vi "Trav_cluster_Convert.vi"(4 "Traverse line in":T1 {"Carrier_2 Q (l/min)" format="%#.2f"; "Row Duration (mins)" format="%#.1f"; "Row No" min=0; "Trace Gas Concentration (%)" min=0.0 format="%#_4f"; "Carrier_1 Q (l/min)" format="%#.4f"; "Start X" format="%#.2f"; "Start Y" format="%#.2f"; "Start Z" format="%#.2f"; "End X" format="%#.2f"; "End Y" format="%#.2f"; "End Z" format="%#.2f"; "Tunnel Speed" format="%#.2f"; "Averaging time (mins)" min=0.0 format="%#.2f"}, 5 "Channel Values In":string[](array[string]), 6 "Row Number":i32, 7 "Channel names":string[](array[string])) -> (0 "Traverse line Out":T1 {"Carrier_2 Q (l/min)" format="%#.2f"; "Row Duration (mins)" format="%#.1f"; "Row No" min=0; "Trace Gas Concentration (%)" min=0.0 format="%#_4f"; "Carrier_1 Q (l/min)" format="%#.4f"; "Start X" format="%#.2f"; "Start Y" format="%#.2f"; "Start Z" format="%#.2f"; "End X" format="%#.2f"; "End Y" format="%#.2f"; "End Z" format="%#.2f"; "Tunnel Speed" format="%#.2f"; "Averaging time (mins)" min=0.0 format="%#.2f"})   [LabVIEW 2020]
uses:
  Traverse_cluster.ctl
  Spacing.ctl
  Controls/Multi_run_mode.ctl
panel:
  # "X           Y          Z"
  # "Start"
  # "End"
  # "X           Y          Z"
  # "Start"
  # "End"
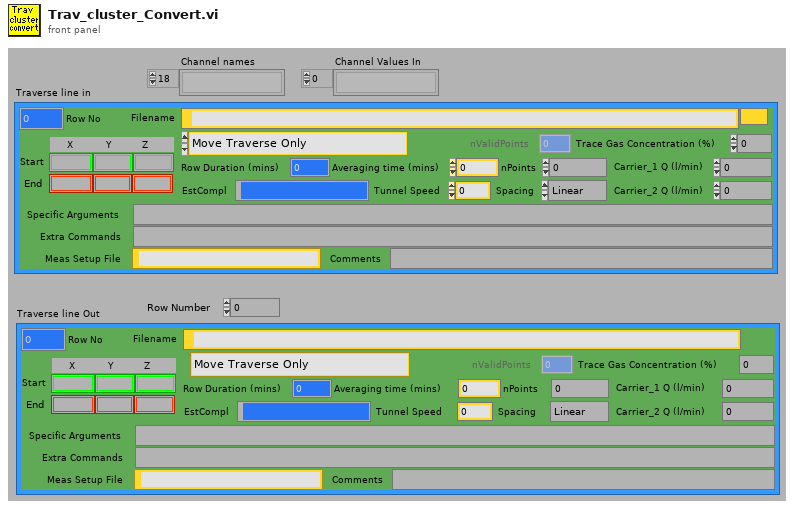
[diagram p1: front panel]
types:
  T1 = typedef "Traverse_cluster.ctl" = cluster{"Start X":sgl, "Start Y":sgl, "Start Z":sgl, "End X":sgl, "End Y":sgl, "End Z":sgl, "nPoints":i32, "Spacing":T2, "Filename":path, "Tunnel Speed":dbl, "Averaging time (mins)":dbl, "Extra Commands":string, "Carrier_1 Q (l/min)":dbl, "Carrier_2 Q (l/min)":dbl, "Trace Gas Concentration (%)":dbl, "Specific Arguments":string, "Comments":string, "Row No":i32, "Row Type Selector":T3, "EstCompl":string, "Row Duration (mins)":dbl, "nValidPoints":i32, "Meas Setup File":string}
  T2 = typedef "Spacing.ctl" = enum16{"Linear", "Log", "Gauss", "Specified", "N/A"}
  T3 = typedef "Multi_run_mode.ctl" = enum16{"Move Traverse Only", "Set Tunnel Speed Only", "Set Source Only", "Set Measurement Conditions", "Single Measurement", "Vertical Profile", "Lateral Profile", "Longitudinal Profile", "Multi-Axis Profile", "Explore Volume", "Auto Calibrate", "Meas Fast FID Bkgnd", "Check Beam Power", "Scanning Valve Measurement", "Run VI Named:", "Set ADAM Ch", "Wait (minutes)", "Send Message", "Synchronize With:", "Fall Back to this Row", "Turn Off Row Repeating", "Traverse 3D Volume", "Blank Row", "Jump to Fall Back Row"}
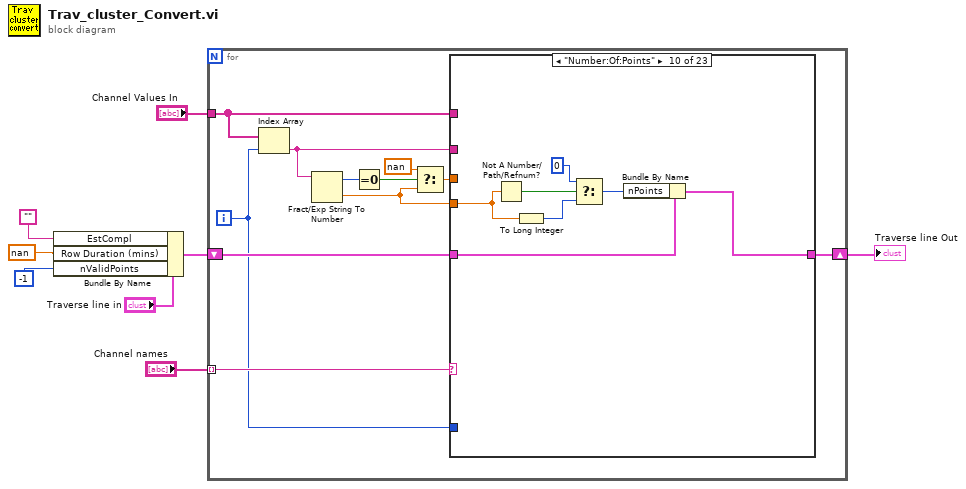
[diagram p0: block diagram]
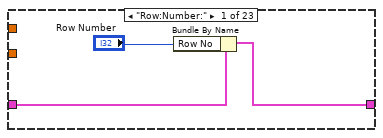
[diagram p2: hidden frame]
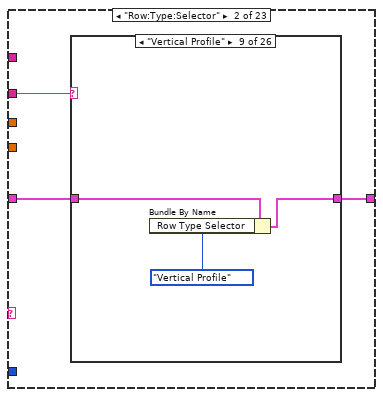
[diagram p3: hidden frame]
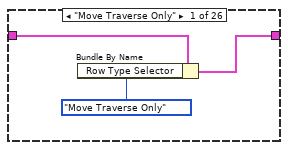
[diagram p4: hidden frame]
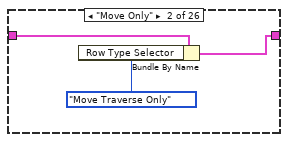
[diagram p5: hidden frame]
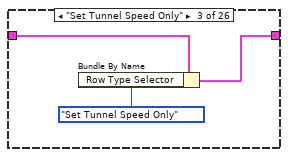
[diagram p6: hidden frame]
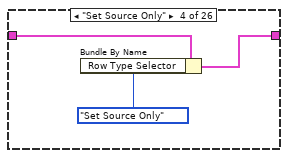
[diagram p7: hidden frame]
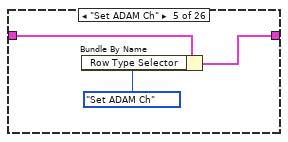
[diagram p8: hidden frame]
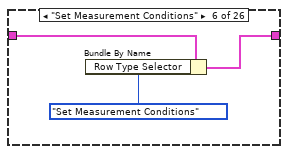
[diagram p9: hidden frame]
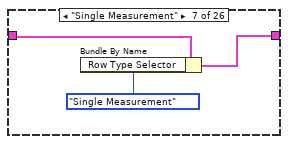
[diagram p10: hidden frame]
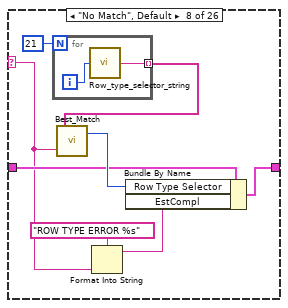
[diagram p11: hidden frame]
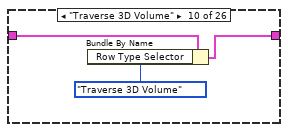
[diagram p12: hidden frame]
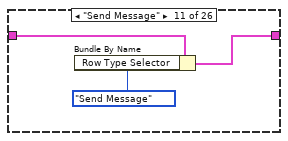
[diagram p13: hidden frame]
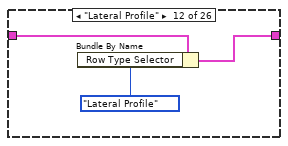
[diagram p14: hidden frame]
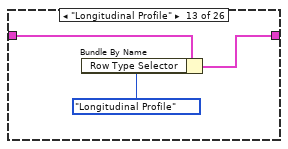
[diagram p15: hidden frame]
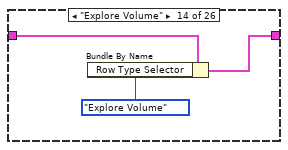
[diagram p16: hidden frame]
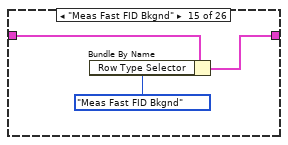
[diagram p17: hidden frame]
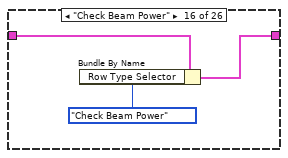
[diagram p18: hidden frame]
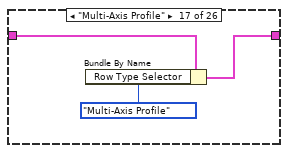
[diagram p19: hidden frame]
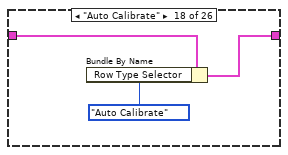
[diagram p20: hidden frame]
diagram:
  n1 = Bundle By Name(cluster="Traverse line in", "EstCompl"="", "Row Duration (mins)"=nan ("Bundle Element"), "nValidPoints"=-1 ("No. of Valid pts.")) -> (w4:T1)
  n2 = for {
    tunnel: "Channel names" -> [w13] mode=indexing
    shift-right: [w18] -> w3
    shift-left: w4 -> [w19]
    tunnel: "Channel Values In" -> [w10]
    i -> [w11]
    n3 = Index Array(array=w10, index=w11) -> (element=w12:string)
    n4 = Fract/Exp String To Number(string=w12) -> (offset past number=w17:i32, number=w9:dbl)  [unwired: 1 in, 2 out]
    n5 = Equal To 0?(x=w17) -> (x = 0?=w16:bool)
    n6 = Select(t=nan ("f"), s=w16, f=w9) -> (s? t:f=w15:dbl)
    n7 = case shown="\"Number:Of:Points\"" w13 {
      selector: w13 -> [_ _ _ _ _ _ _ _ _ _ _ _ _ _ _ _ _ _ _ _ _ _ w184]
      tunnel: w19 -> [w21 w24 w112 w115 w118 w122 w125 w127 w130 w132 w142 w148 w151 w156 w160 w163 w164 w167 w170 w176 w182 w183 w185]
      tunnel: w9 -> [_ _ _ _ _ _ _ _ _ w135 _ w147 _ _ _ _ w166 w169 w172 _ _ _ _]
      tunnel: [w22 w23 w113 w116 w119 w121 w124 w128 w131 w138 w141 w149 w154 w157 w159 w162 w165 w168 w171 w178 w182 w183 w185] -> w18
      tunnel: w12 -> [_ w25 _ _ _ _ _ _ _ _ w140 _ w153 w155 w158 w161 _ _ _ w175 _ _ _]
      tunnel: w11 -> [_ _ _ _ _ _ _ _ _ _ _ _ _ _ _ _ _ _ _ _ _ _ _]
      tunnel: w15 -> [_ _ w111 w114 w117 w120 w123 w126 w129 _ _ _ _ _ _ _ _ _ _ _ _ _ _]
      tunnel: w10 -> [_ _ _ _ _ _ _ _ _ _ _ _ _ _ _ _ _ _ _ w173 _ _ _]
      frame "Row:Number:" {
        n8 = Bundle By Name(cluster=w21, "Row No"="Row Number") -> (w22:T1)
      }
      frame "Row:Type:Selector" {
        n9 = case shown="\"Vertical Profile\"" w25 {
          selector: w25 -> [_ _ _ _ _ _ _ w47 _ _ _ _ _ _ _ _ _ _ _ _ _ _ _ _ _ _]
          tunnel: w24 -> [w28 w30 w33 w36 w39 w42 w45 w51 w58 w61 w64 w68 w70 w74 w76 w79 w82 w86 w88 w91 w94 w97 w100 w103 w106 w109]
          tunnel: [w27 w29 w32 w35 w38 w41 w44 w50 w59 w62 w63 w67 w69 w72 w75 w78 w81 w85 w87 w90 w93 w96 w99 w102 w107 w110] -> w23
          frame "Move Traverse Only" {
            n10 = Bundle By Name(cluster=w28, "Row Type Selector"=Multi_run_mode."Move Traverse Only" ("Mode")) -> (w27:T1)
          }
          frame "Move Only" {
            n11 = Bundle By Name(cluster=w30, "Row Type Selector"=Multi_run_mode."Move Traverse Only" ("Mode")) -> (w29:T1)
          }
          frame "Set Tunnel Speed Only" {
            n12 = Bundle By Name(cluster=w33, "Row Type Selector"=Multi_run_mode."Set Tunnel Speed Only" ("Mode")) -> (w32:T1)
          }
          frame "Set Source Only" {
            n13 = Bundle By Name(cluster=w36, "Row Type Selector"=Multi_run_mode."Set Source Only" ("Mode")) -> (w35:T1)
          }
          frame "Set ADAM Ch" {
            n14 = Bundle By Name(cluster=w39, "Row Type Selector"=Multi_run_mode."Set ADAM Ch" ("Mode")) -> (w38:T1)
          }
          frame "Set Measurement Conditions" {
            n15 = Bundle By Name(cluster=w42, "Row Type Selector"=Multi_run_mode."Set Measurement Conditions" ("Mode")) -> (w41:T1)
          }
          frame "Single Measurement" {
            n16 = Bundle By Name(cluster=w45, "Row Type Selector"=Multi_run_mode."Single Measurement" ("Mode")) -> (w44:T1)
          }
          frame "No Match", Default {
            n17 = for {
              N: 21 -> [_]
              tunnel: [w55] -> w53 mode=indexing
              i -> [w56]
              n18 = call "Row_type_selector_string.vi"("Mode"=w56) -> ("Output string"=w55:string)
            }
            n19 = call "Best_Match.vi"("Input String"=w47, "String Options"=w53) -> ("index of element"=w52:i32)  [unwired: 1 out]
            n20 = Format Into String(format string="ROW TYPE ERROR %s", w47) -> (resulting string=w48:string)  [unwired: 2 in, 1 out]
            n21 = Bundle By Name(cluster=w51, "Row Type Selector"=w52, "EstCompl"=w48) -> (w50:T1)
          }
          frame "Vertical Profile" {
            n22 = Bundle By Name(cluster=w58, "Row Type Selector"=Multi_run_mode."Vertical Profile" ("Mode")) -> (w59:T1)
          }
          frame "Traverse 3D Volume" {
            n23 = Bundle By Name(cluster=w61, "Row Type Selector"=Multi_run_mode."Traverse 3D Volume" ("Mode")) -> (w62:T1)
          }
          frame "Send Message" {
            n24 = Bundle By Name(cluster=w64, "Row Type Selector"=Multi_run_mode."Send Message" ("Mode")) -> (w63:T1)
          }
          frame "Lateral Profile" {
            n25 = Bundle By Name(cluster=w68, "Row Type Selector"=Multi_run_mode."Lateral Profile" ("Mode")) -> (w67:T1)
          }
          frame "Longitudinal Profile" {
            n26 = Bundle By Name(cluster=w70, "Row Type Selector"=Multi_run_mode."Longitudinal Profile" ("Mode")) -> (w69:T1)
          }
          frame "Explore Volume" {
            n27 = Bundle By Name(cluster=w74, "Row Type Selector"=Multi_run_mode."Explore Volume" ("Mode")) -> (w72:T1)
          }
          frame "Meas Fast FID Bkgnd" {
            n28 = Bundle By Name(cluster=w76, "Row Type Selector"=Multi_run_mode."Meas Fast FID Bkgnd" ("Mode")) -> (w75:T1)
          }
          frame "Check Beam Power" {
            n29 = Bundle By Name(cluster=w79, "Row Type Selector"=Multi_run_mode."Check Beam Power" ("Mode")) -> (w78:T1)
          }
          frame "Multi-Axis Profile" {
            n30 = Bundle By Name(cluster=w82, "Row Type Selector"=Multi_run_mode."Multi-Axis Profile" ("Mode")) -> (w81:T1)
          }
          frame "Auto Calibrate" {
            n31 = Bundle By Name(cluster=w86, "Row Type Selector"=Multi_run_mode."Auto Calibrate" ("Mode")) -> (w85:T1)
          }
          frame "Scanning Valve Measurement" {
            n32 = Bundle By Name(cluster=w88, "Row Type Selector"=Multi_run_mode."Scanning Valve Measurement" ("Mode")) -> (w87:T1)
          }
          frame "Wait (minutes)" {
            n33 = Bundle By Name(cluster=w91, "Row Type Selector"=Multi_run_mode."Wait (minutes)" ("Mode")) -> (w90:T1)
          }
          frame "Run VI Named:" {
            n34 = Bundle By Name(cluster=w94, "Row Type Selector"=Multi_run_mode."Run VI Named:" ("Mode")) -> (w93:T1)
          }
          frame "Synchronize With:" {
            n35 = Bundle By Name(cluster=w97, "Row Type Selector"=Multi_run_mode."Synchronize With:" ("Mode")) -> (w96:T1)
          }
          frame "Fall Back to this Row" {
            n36 = Bundle By Name(cluster=w100, "Row Type Selector"=Multi_run_mode."Fall Back to this Row" ("Mode")) -> (w99:T1)
          }
          frame "Turn Off Row Repeating" {
            n37 = Bundle By Name(cluster=w103, "Row Type Selector"=Multi_run_mode."Turn Off Row Repeating" ("Mode")) -> (w102:T1)
          }
          frame "" {
            n38 = Bundle By Name(cluster=w106, "Row Type Selector"=Multi_run_mode."Blank Row" ("Mode")) -> (w107:T1)
          }
          frame "Jump to Fall Back Row" {
            n39 = Bundle By Name(cluster=w109, "Row Type Selector"=Multi_run_mode."Blank Row" ("Mode")) -> (w110:T1)
          }
        }
      }
      frame "Tunnel:Speed:(m/s)" {
        n40 = Bundle By Name(cluster=w112, "Tunnel Speed"=w111) -> (w113:T1)
      }
      frame "Start at:X:(mm)" {
        n41 = Bundle By Name(cluster=w115, "Start X"=w114) -> (w116:T1)
      }
      frame "Start at:Y:(mm)" {
        n42 = Bundle By Name(cluster=w118, "Start Y"=w117) -> (w119:T1)
      }
      frame "Start at:Z:(mm)" {
        n43 = Bundle By Name(cluster=w122, "Start Z"=w120) -> (w121:T1)
      }
      frame "End at:X:(mm)" {
        n44 = Bundle By Name(cluster=w125, "End X"=w123) -> (w124:T1)
      }
      frame "End at:Y:(mm)" {
        n45 = Bundle By Name(cluster=w127, "End Y"=w126) -> (w128:T1)
      }
      frame "End at:Z:(mm)" {
        n46 = Bundle By Name(cluster=w130, "End Z"=w129) -> (w131:T1)
      }
      frame "Number:Of:Points" {
        n47 = Not A Number/Path/Refnum?(number/path/refnum=w135) -> (NaN/Path/Refnum?=w137:bool)
        n48 = To Long Integer(number=w135) -> (32bit integer=w136:i32)
        n49 = Select(t=0, s=w137, f=w136) -> (s? t:f=w133:i32)
        n50 = Bundle By Name(cluster=w132, "nPoints"=w133) -> (w138:T1)
      }
      frame "Point:Spacing:Method" {
        n51 = case shown="\"Linear\", Default" w140 {
          tunnel: [Spacing."Linear" ("Spacing") Spacing."Log" ("Spacing") Spacing."Gauss" ("Spacing") Spacing."Specified" ("Spacing")] -> w139
          frame "Linear", Default {
          }
          frame "Log" {
          }
          frame "Gauss" {
          }
          frame "Specified" {
          }
        }
        n52 = Bundle By Name(cluster=w142, "Spacing"=w139) -> (w141:T1)
      }
      frame "Averaging:Time:(mins)" {
        n53 = Bundle By Name(cluster=w148, "Averaging time (mins)"=w147) -> (w149:T1)
      }
      frame "Filename:HD:Users" {
        n54 = call "Text_without_format.vi"("Input string"=w153) -> ("Output string"=w152:string)
        n55 = String To Path(string=w152) -> (path=w150:path)
        n56 = Bundle By Name(cluster=w151, "Filename"=w150) -> (w154:T1)
      }
      frame "Specific:Arguments:String" {
        n57 = Bundle By Name(cluster=w156, "Specific Arguments"=w155) -> (w157:T1)
      }
      frame "Measurement:Setup:File" {
        n58 = Bundle By Name(cluster=w160, "Meas Setup File"=w158) -> (w159:T1)
      }
      frame "Extra:Commands:String" {
        n59 = Bundle By Name(cluster=w163, "Extra Commands"=w161) -> (w162:T1)
      }
      frame "Carrier_1:Q:(l/min)" {
        n60 = Bundle By Name(cluster=w164, "Carrier_1 Q (l/min)"=w166) -> (w165:T1)
      }
      frame "Carrier_2:Q:(l/min)" {
        n61 = Bundle By Name(cluster=w167, "Carrier_2 Q (l/min)"=w169) -> (w168:T1)
      }
      frame "Trace Gas:Concentration:(%)" {
        n62 = Bundle By Name(cluster=w170, "Trace Gas Concentration (%)"=w172) -> (w171:T1)
      }
      frame "Comments::" {
        n63 = Unbundle By Name(w176) -> ("Row Type Selector"=w177:T3)
        n64 = case shown="\"Set ADAM Ch\", Default" w177 {
          tunnel: [w179 w180] -> w174
          tunnel: w175 -> [w179 _]
          tunnel: w173 -> [_ w181]
          frame "Set ADAM Ch", Default {
          }
          frame "Blank Row" {
            n65 = Concatenate Strings(w181) -> (w180:string)
          }
        }
        n66 = Bundle By Name(cluster=w176, "Comments"=w174) -> (w178:T1)
      }
      frame "Row:Completion:Time" {
      }
      frame "Time:Taken in:Row (mins)" {
      }
      frame "No match", Default {
        n67 = call "Was_string_matched.vi"("Variable name"=w184) -> ()  [unwired: 2 in]
      }
    }
  }
  "Traverse line Out" <- w3
